vi "zero control.vi"(6 "Valve control":bool=TRUE, 7 "Ctl Refnum":refnum<vi>, 8 "error in (no error)":errorcluster, 9 "Zero now":bool, 10 "Zero timer":bool, 11 "VISA resource name":refnum<visa-resource-name>) -> (0 "error out":errorcluster, 1 "Zero reset":bool, 3 "VISA resource out":refnum<visa-resource-name>)   [LabVIEW 2016]
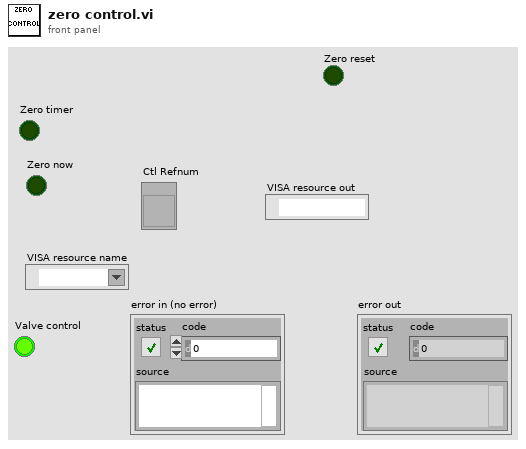
[diagram p1: front panel]
types:
  T1 = enum16{"Time", "Zero", "Poll", "Read Buffer", "Set Stream", "Set Poll", "Pump On", "Pump Off", "Set Zero Timing", "Set CO2 Avg.", "Set Measument Format", "Startup Zero Off", "Statup Zero On", "Short Zero Duration", "Set Scaling Factor", "Set Dec Points", "Set Low CO2 Alarm", "Set Analog Output Type", "Set Analog Output Scaling", "Set Data Valid Pin I/O", "Save Current Settings", "Restore Default Settings", "Display Current Settings", "Medium Zero Duration", "Long Zero Duration"}
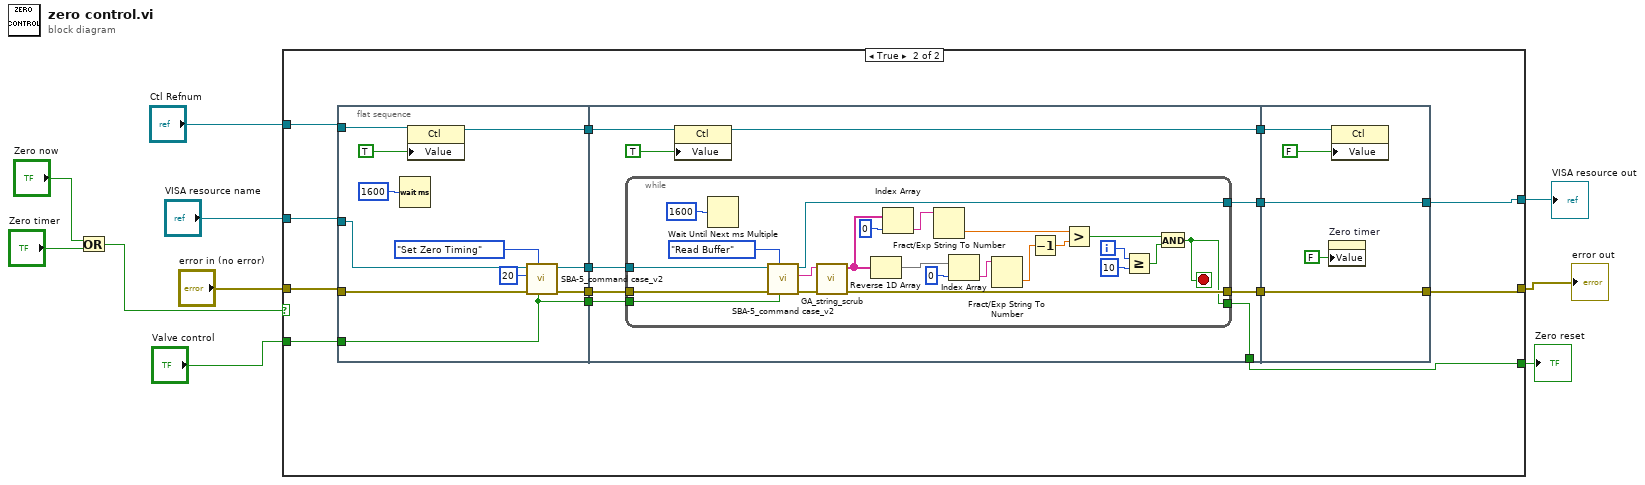
[diagram p0: block diagram]
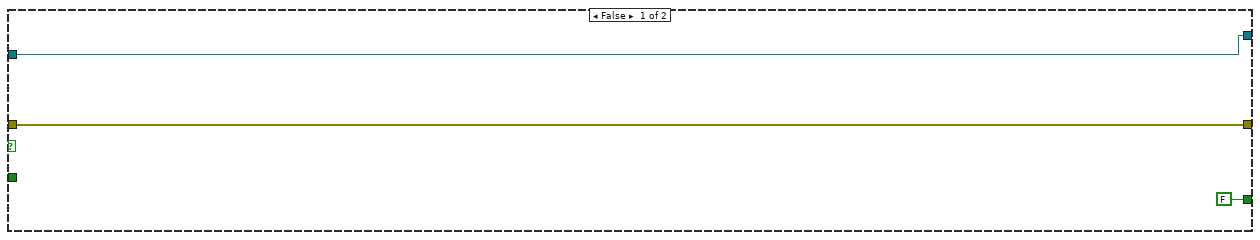
[diagram p2: hidden frame]
diagram:
  n1 = Or(x="Zero now", y="Zero timer") -> (x .or. y?=w2:bool)
  n2 = case shown="True" w2 {
    tunnel: "error in (no error)" -> [w13 w21]
    tunnel: [w13 w17] -> w6
    tunnel: [w11 w18] -> w5
    tunnel: [FALSE w16] -> w4
    tunnel: "VISA resource name" -> [w11 w20]
    tunnel: "Ctl Refnum" -> [_ w19]
    tunnel: "Valve control" -> [_ w15]
    frame False {
    }
    frame True {
      n3 = flat-sequence {
        tunnel: w21 -> [w36]
        tunnel: w20 -> [w35]
        tunnel: [w34] -> w27
        tunnel: [w33] -> w26
        tunnel: w19 -> [w31]
        tunnel: [w30] -> w25
        tunnel: w15 -> [w28]
        tunnel: [w28] -> w14
        tunnel: [w45] -> w16
        tunnel: [w47] -> w24
        tunnel: [w46] -> w23
        tunnel: w27 -> [w43]
        tunnel: w26 -> [w42]
        tunnel: w25 -> [w41]
        tunnel: [w40] -> w22
        tunnel: w14 -> [w39]
        tunnel: [w74] -> w17
        tunnel: [w75] -> w18
        tunnel: w24 -> [w75]
        tunnel: w23 -> [w74]
        tunnel: w22 -> [w72]
        frame #0 {
          n4 = Wait (ms)(milliseconds to wait=u32 1600) -> ()  [unwired: 1 out]
          n5 = property on="Property Node" class="Ctl"(reference=w31, "Value"=TRUE) -> (reference out=w30:refnum<vi>)  [unwired: 1 in, 1 out]
          n6 = call "SBA-5_command case_v2.vi"("Valve control"=w28, "Case"=T1."Set Zero Timing", "error in (no error)"=w36, "Val 1"=20, "VISA resource name"=w35) -> ("error out"=w33:errorcluster, "dup VISA resource name"=w34:refnum<visa-resource-name>)  [unwired: 3 in, 2 out]
        }
        frame #1 {
          n7 = while {
            tunnel: [w52] -> w47
            tunnel: [w70] -> w46
            tunnel: [w63] -> w45
            tunnel: w43 -> [w54]
            tunnel: w42 -> [w53]
            tunnel: w39 -> [w48]
            i -> [w57]
            stop <- w63 stop-if-true
            n8 = Wait Until Next ms Multiple(millisecond multiple=u32 1600) -> ()  [unwired: 1 out]
            n9 = call "SBA-5_command case_v2.vi"("Valve control"=w48, "Case"=T1."Read Buffer", "error in (no error)"=w53, "VISA resource name"=w54) -> ("error out"=w51:errorcluster, "StringFromSBA-5"=w50:string, "dup VISA resource name"=w52:refnum<visa-resource-name>)  [unwired: 4 in, 1 out]
            n10 = call "GA_string_scrub.vi"("error in (no error)"=w51, "input"=w50) -> ("error out"=w70:errorcluster, "output array"=w68:string[])  [unwired: 2 in, 6 out]
            n11 = Reverse 1D Array(array=w68) -> (reversed array=w69:string[])
            n12 = Index Array(array=w68, index=0) -> (element=w65:string)
            n13 = Fract/Exp String To Number(string=w65) -> (number=w62:dbl)  [unwired: 3 in, 1 out]
            n14 = Index Array(array=w69, index=0) -> (element=w64:string)
            n15 = Fract/Exp String To Number(string=w64) -> (number=w61:dbl)  [unwired: 3 in, 1 out]
            n16 = Decrement(x=w61) -> (x-1=w60:dbl)
            n17 = Greater?(x=w62, y=w60) -> (0:w59:bool)
            n18 = Greater Or Equal?(x=w57, y=10) -> (x >= y?=w58:bool)
            n19 = And(x=w59, y=w58) -> (x .and. y?=w63:bool)
          }
          n20 = property on="Property Node" class="Ctl"(reference=w41, "Value"=TRUE) -> (reference out=w40:refnum<vi>)  [unwired: 1 in, 1 out]
        }
        frame #2 {
          n21 = property on="Zero timer" class="Bool (strict)"("Value"=FALSE ("Zero timer")) -> ()  [unwired: 2 in, 2 out]
          n22 = property on="Property Node" class="Ctl"(reference=w72, "Value"=FALSE) -> ()  [unwired: 1 in, 2 out]
        }
      }
    }
  }
  "VISA resource out" <- w5
  "error out" <- w6
  "Zero reset" <- w4
